vi "基本比较器（dbl[]）.vi"(0 "输入":dbl[](array[numeric]), 1 "基准":dbl[](array[numeric])) -> (2 "大于":bool, 3 "等于":bool, 4 "小于":bool)   [LabVIEW 2012]
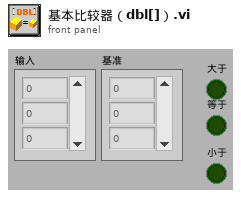
[diagram p1: front panel]
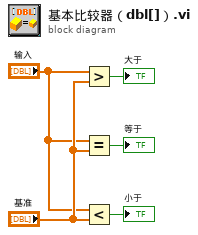
[diagram p0: block diagram]
diagram:
  n1 = Greater?(x="输入", y="基准") -> (0:→"大于":bool)
  n2 = Equal?(x="输入", y="基准") -> (x = y?=→"等于":bool)
  n3 = Less?(x="输入", y="基准") -> (x < y?=→"小于":bool)
